vi "流程固件设置对话框.vi"() -> ()   [LabVIEW 2016, in "斯坦道氨氮.lvlib"]
uses:
  <vilib>/Utility/miscctls.llb/LVPointTypeDef.ctl
panel:
  in  "修改系列号":bool
  in  "关闭":bool
  in  "外设设置":bool
  in  "固件升级":bool
  in  "流程写入":bool
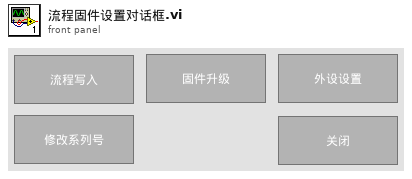
[diagram p1: front panel]
types:
  T1 = enum32{"Invalid", "Standard", "Closed", "Hidden", "Minimized", "Maximized"}
  T2 = typedef "LVPointTypeDef.ctl" = cluster{"Horizontal":i16, "Vertical":i16}
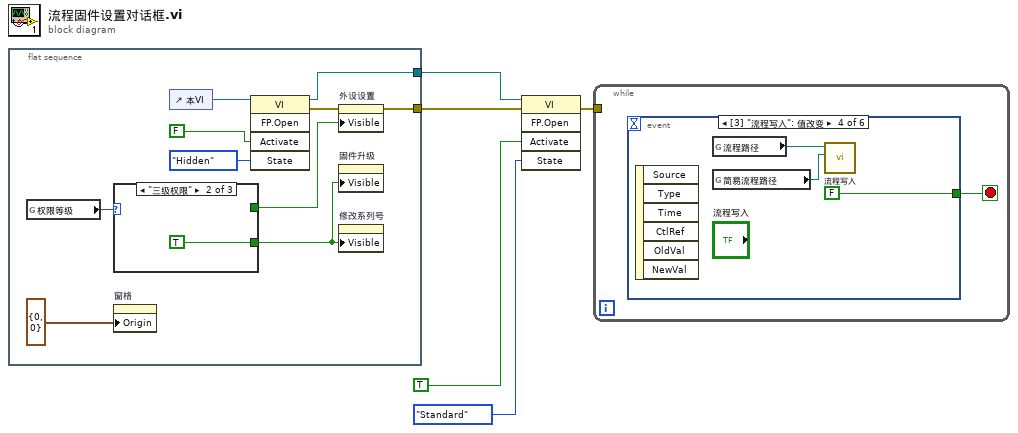
[diagram p0: block diagram]
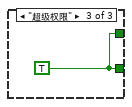
[diagram p3: hidden frame]
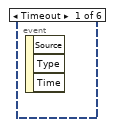
[diagram p4: hidden frame]
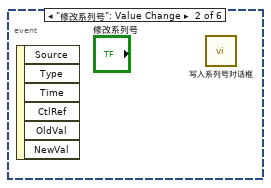
[diagram p5: hidden frame]
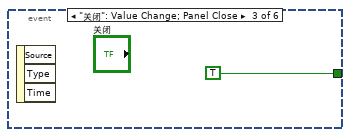
[diagram p6: hidden frame]
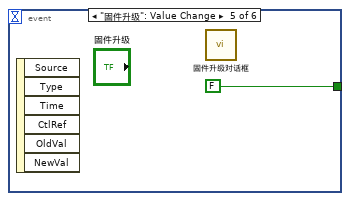
[diagram p7: hidden frame]
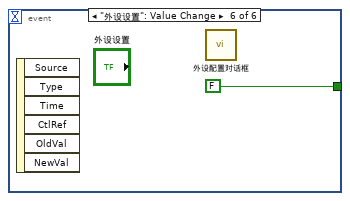
[diagram p8: hidden frame]
diagram:
  n1 = flat-sequence {
    tunnel: [w8] -> w5
    tunnel: [w7] -> w4
    frame #0 {
      n2 = global read "VAR总磷总氮全局变量.vi" "权限等级"() -> (w14:enum16{"一级权限", "二级权限", "三级权限", "超级权限"})
      n3 = case shown="\"三级权限\"" w14 {
        tunnel: [_ TRUE w17] -> w12
        tunnel: [_ _ w17] -> w13
        frame "一级权限", Default {
        }
        frame "三级权限" {
        }
        frame "超级权限" {
          w17 = TRUE
        }
      }
      n4 = property on="窗格" class="Pane"("Origin"=T2 {"Horizontal"=0, "Vertical"=0} ("原点")) -> ()  [unwired: 2 in, 2 out]
      n5 = control-ref of="本VI"() -> (w11:refnum<vi>)
      n6 = invoke class="VI" method="FP.Open"(reference=w11, "Activate"=FALSE ("激活？"), "State"=T1."Hidden" ("状态")) -> (reference out=w8:refnum<vi>, error out=w9:errorcluster)  [unwired: 2 in, 3 out]
      n7 = property on="外设设置" class="Bool"(error in=w9, "Visible"=w13) -> (error out=w7:errorcluster)  [unwired: 1 in, 1 out]
      n8 = property on="固件升级" class="Bool"("Visible"=w12) -> ()  [unwired: 2 in, 2 out]
      n9 = property on="修改系列号" class="Bool"("Visible"=w12) -> ()  [unwired: 2 in, 2 out]
    }
  }
  n10 = invoke class="VI" method="FP.Open"(reference=w5, error in=w4, "Activate"=TRUE ("激活？"), "State"=T1."Standard" ("状态")) -> (error out=w1:errorcluster)  [unwired: 1 in, 4 out]
  n11 = while {
    tunnel: w1 -> [_]
    stop <- w18 stop-if-true
    n12 = event shown="[3] \"流程写入\": 值改变" {
      selector: _ -> [_ _ _ _ _ _]
      dyn-events: _ -> [_ _ _ _ _ _]
      timeout: _ -> [_ _ _ _ _ _]
      tunnel: [_ _ TRUE FALSE FALSE FALSE] -> w18
      event Timeout {
        n13 = event-data() -> ()  [unwired: 1 in, 3 out]
      }
      event "修改系列号": Value Change {
        n14 = event-data() -> ()  [unwired: 1 in, 6 out]
        n15 = call "写入系列号对话框.vi"() -> ()  [unwired: 12 in]
      }
      event "关闭": Value Change; Panel Close {
        n16 = event-data() -> ()  [unwired: 1 in, 3 out]
      }
      event "流程写入": Value Change {
        n17 = event-data() -> ()  [unwired: 1 in, 6 out]
        n18 = global read "总磷总氮断电保存全局变量.vi" "流程路径"() -> (w21:path)
        n19 = global read "总磷总氮断电保存全局变量.vi" "简易流程路径"() -> (w20:path)
        n20 = call "流程写入.vi"("简易流程路径"=w20, "添加的路径"=w21) -> ()  [unwired: 10 in]
      }
      event "固件升级": Value Change {
        n21 = event-data() -> ()  [unwired: 1 in, 6 out]
        n22 = call "固件升级对话框.vi"() -> ()  [unwired: 12 in]
      }
      event "外设设置": Value Change {
        n23 = event-data() -> ()  [unwired: 1 in, 6 out]
        n24 = call "外设配置对话框.vi"() -> ()  [unwired: 12 in]
      }
    }
  }
